vi "ATF-Pump-Flush Queue.vi"(8 "error in (no error)":errorcluster, 11 "Data FIFO Ref":T1) -> (0 "error out":errorcluster)   [LabVIEW 2022 SP3]
uses:
  RT Controls/ATF-Pump-Data FIFO.ctl
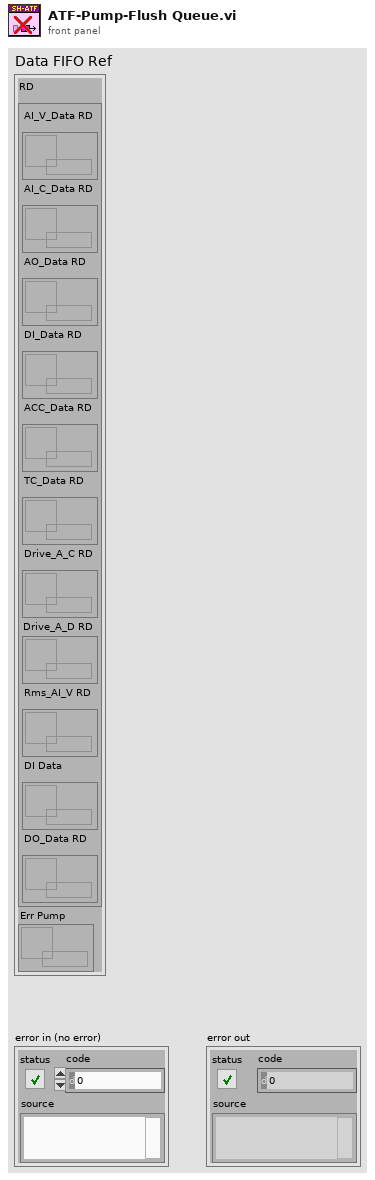
[diagram p1: front panel]
types:
  T1 = typedef "ATF-Pump-Data FIFO.ctl" = cluster{"RD":cluster{"AI_V_Data RD":refnum<queue>, "AI_C_Data RD":refnum<queue>, "AO_Data RD":refnum<queue>, "DI_Data RD":refnum<queue>, "ACC_Data RD":refnum<queue>, "TC_Data RD":refnum<queue>, "Drive_A_C RD":refnum<queue>, "Drive_A_D RD":refnum<queue>, "Rms_AI_V RD":refnum<queue>, "DI Data":refnum<queue>, "DO_Data RD":refnum<queue>}, "Err Pump":refnum<queue>}
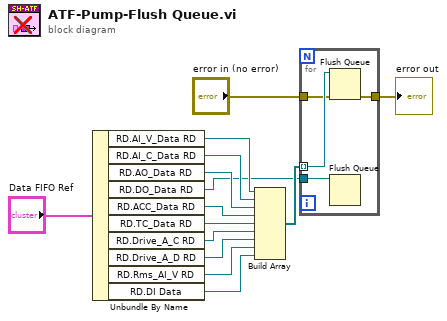
[diagram p0: block diagram]
diagram:
  n1 = Unbundle By Name("Data FIFO Ref") -> ("RD.AI_V_Data RD"=w13:refnum<queue>, "RD.AI_C_Data RD"=w12:refnum<queue>, "RD.AO_Data RD"=w11:refnum<queue>, "RD.DO_Data RD"=w1:refnum<queue>, "RD.ACC_Data RD"=w10:refnum<queue>, "RD.TC_Data RD"=w9:refnum<queue>, "RD.Drive_A_C RD"=w8:refnum<queue>, "RD.Drive_A_D RD"=w7:refnum<queue>, "RD.Rms_AI_V RD"=w6:refnum<queue>, "RD.DI Data"=w5:refnum<queue>)
  n2 = Build Array(w13, w12, w11, w10, w9, w8, w7, w6, w5) -> (w4:refnum<queue>[])
  n3 = for {
    tunnel: w4 -> [w18] mode=indexing
    tunnel: "error in (no error)" -> [w17]
    tunnel: [w16] -> w2
    tunnel: w1 -> [w15]
    n4 = Flush Queue(queue=w18, error in (no error)=w17) -> (error out=w16:errorcluster)  [unwired: 2 out]
    n5 = Flush Queue(queue=w15) -> ()  [unwired: 1 in, 3 out]
  }
  "error out" <- w2
